vi "FPGA_Incremental_Enc_Port_Forward.vi"() -> ()   [LabVIEW 2019]
uses:
  <vilib>/rvi/Emulation/niFpgaSctlEmulationGetInTimedLoop.vi
  <vilib>/rvi/Emulation/niFpgaProcessEmulError.vi
  <vilib>/rvi/Emulation/niFpgaGetClockAttributes.vi
  <vilib>/rvi/Emulation/niFpgaEmulationReportErrorSimple.vi
  <vilib>/rvi/eio/common/nirviEmuTemplateMethod_errors.vi
  <vilib>/rvi/Emulation/niFpgaCriticalErrorInLSC.vi
  <vilib>/eio/EIONode/EIONode.xnode
panel:
  in  "stop":bool
  out "ConnectorA/DIO9":bool
  out "ConnectorA/DIO8":bool
  out "ConnectorA/DIO10":bool
  out "ConnectorA/DIO11":bool
  out "ConnectorA/DIO13":bool
  out "ConnectorA/DIO12":bool
  out "ConnectorA/DIO15":bool
  out "ConnectorA/DIO14":bool
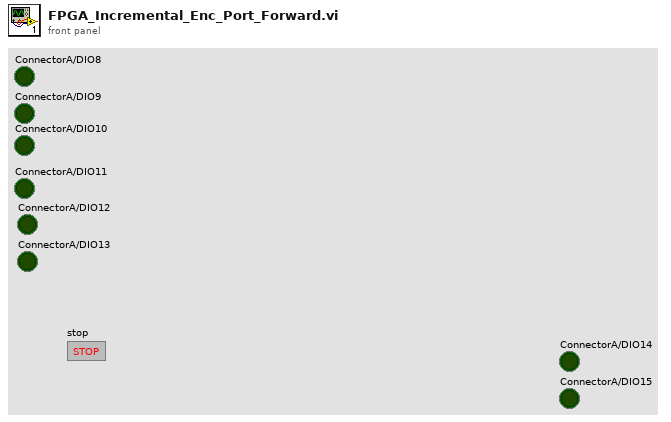
[diagram p1: front panel]
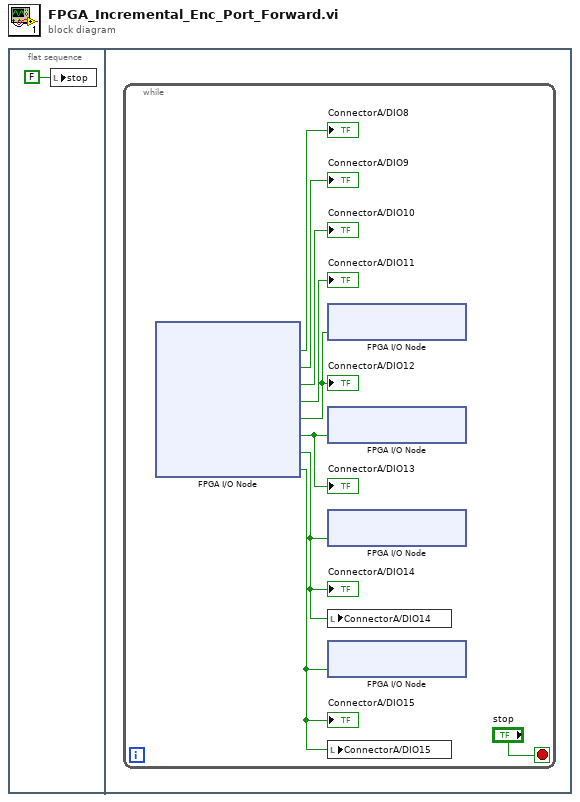
[diagram p0: block diagram]
diagram:
  n1 = flat-sequence {
    frame #0 {
      n2 = local write "stop"(FALSE ("stop")) -> ()
    }
    frame #1 {
      n3 = while {
        stop <- "stop" stop-if-true
        n4 = xnode "FPGA I/O Node"() -> ("ConnectorA/DIO8"=→"ConnectorA/DIO8":bool, "ConnectorA/DIO9"=→"ConnectorA/DIO9":bool, "ConnectorA/DIO10"=→"ConnectorA/DIO10":bool, "ConnectorA/DIO11"=→"ConnectorA/DIO11":bool, "ConnectorA/DIO12"=w4:bool, "ConnectorA/DIO13"=w3:bool, "ConnectorA/DIO14"=w6:bool, "ConnectorA/DIO15"=w5:bool)  [unwired: 8 in, 8 out]
        "ConnectorA/DIO14" <- w6
        "ConnectorA/DIO15" <- w5
        "ConnectorA/DIO12" <- w4
        "ConnectorA/DIO13" <- w3
        n5 = xnode "FPGA I/O Node"("ConnectorA/DIO2"=w4) -> ()  [unwired: 1 in, 1 out]
        n6 = xnode "FPGA I/O Node"("ConnectorA/DIO3"=w3) -> ()  [unwired: 1 in, 1 out]
        n7 = xnode "FPGA I/O Node"("ConnectorA/DIO1"=w6) -> ()  [unwired: 1 in, 1 out]
        n8 = local write "ConnectorA/DIO14"(w6) -> ()
        n9 = xnode "FPGA I/O Node"("ConnectorA/DIO0"=w5) -> ()  [unwired: 1 in, 1 out]
        n10 = local write "ConnectorA/DIO15"(w5) -> ()
      }
    }
  }
